vi "S8300E_SATA_IF_TEST_WIH.vi"() -> ()   [LabVIEW 2011]
panel:
  out "PRELOG2":string
  out "PRELOG1":string
  out "SATA_HDD_SIZE":string
  out "CMDList":cluster{string, string, string}[](array[cluster])
  out "log msg":string
  out "VISA resource name out":refnum<visa-resource-name>
  out "BEGIN TIME":u32
  out "進行狀況":string
  # "2015-6-1"
  # "S8300E SATA Interface Test(接UART COM9)"
  # "Error Code:SATA-IF"
  # "Step1:Check SATA HDD Size\nStep2:Check SATA HDD Interface"
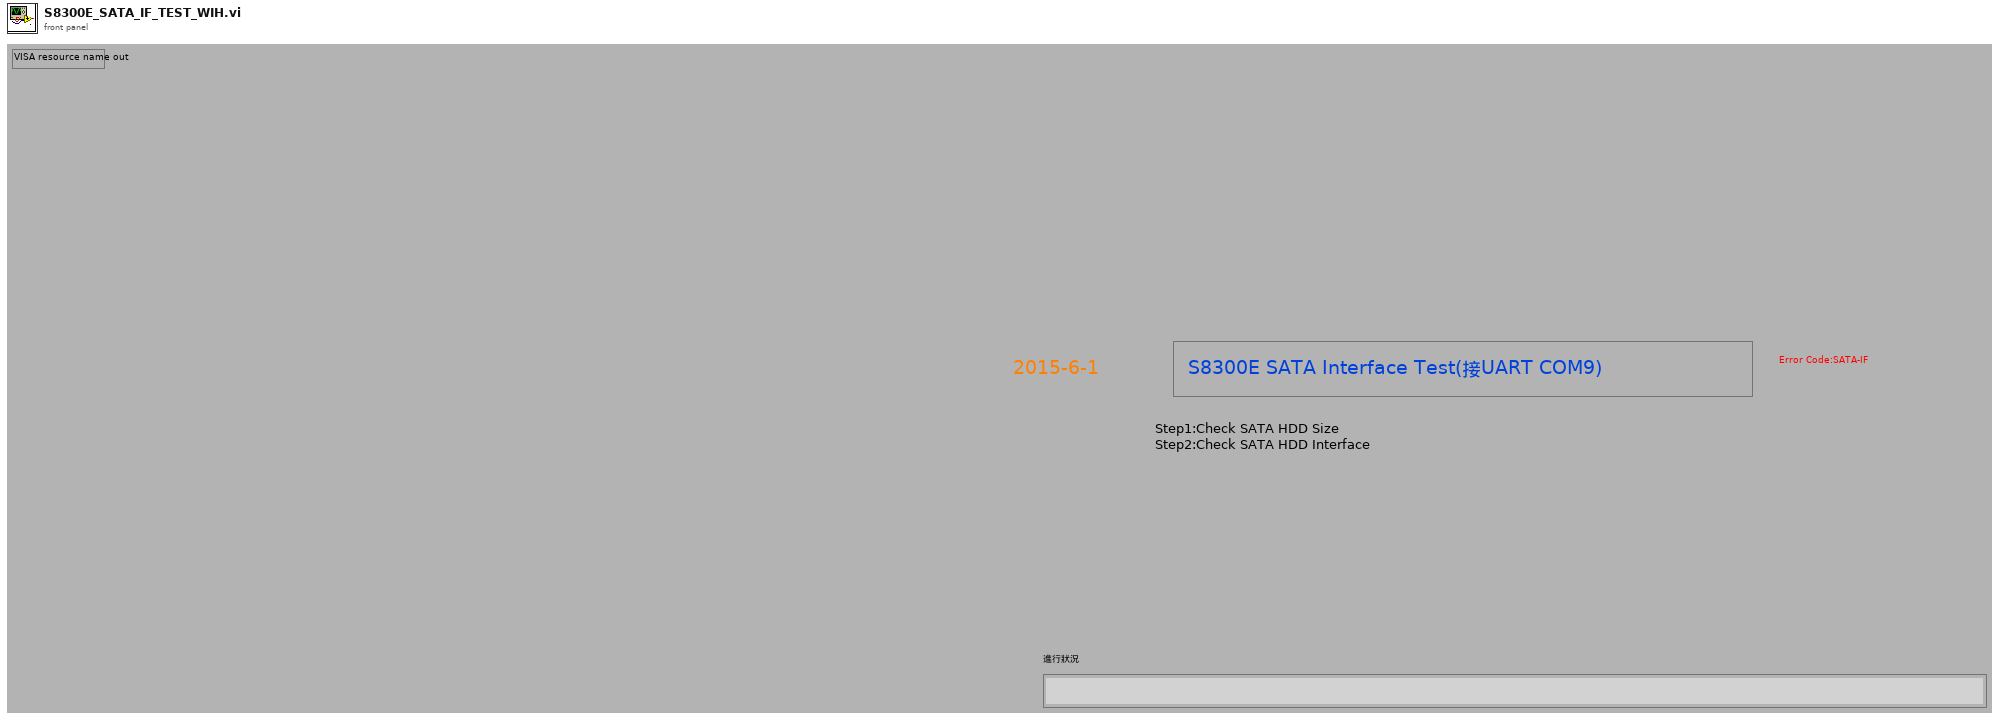
[diagram p1: front panel]
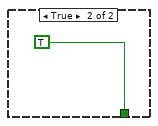
[diagram p7: hidden frame]
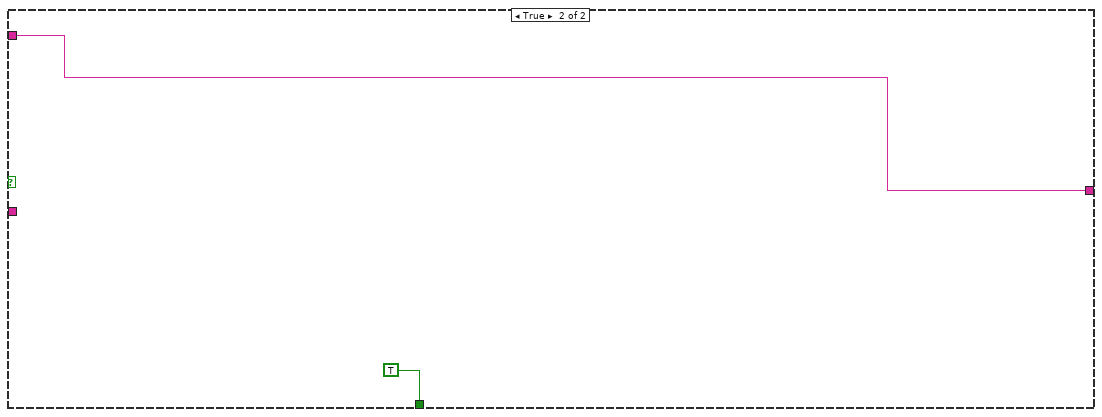
[diagram p9: hidden frame]
diagram:
  n1 = flat-sequence {
    frame #0 {
      n2 = Tick Count (ms)() -> (millisecond timer value=→"BEGIN TIME":u32)
    }
    frame #1 {
      n3 = property on="進行狀況" class="Str"("Blinking"=TRUE) -> ()  [unwired: 2 in, 2 out]
      "進行狀況" <- "進入測試準備中...." ("進行狀況")
    }
    frame #2 {
      n4 = call "SUB_SearchFile_inFolder.vi"("Search Filename in Folder"="S8300E_sfcs_misc.txt") -> ("File Existing True/Flase"=w4:bool)  [unwired: 1 in]
      n5 = case shown="False" w4 {
        frame False {
          n6 = flat-sequence {
            frame #0 {
              n7 = call "Display Message to User"() -> ()  [unwired: 10 in, 2 out]
            }
            frame #1 {
              n8 = call "SUB_Writelog.vi"("Pass/Fail"="Fail:S8300E_SATA_IF_TEST") -> ()  [unwired: 2 in]
            }
            frame #2 {
              n9 = Quit LabVIEW(quit? (T)=TRUE) -> ()
            }
          }
        }
        frame True {
        }
      }
    }
    frame #3 {
      n10 = call "SUB_Read_specifFile.vi"("name or relative path"="S8300E_sfcs_misc.txt" ("Search Filename in Folder")) -> ("text"=w11:string)  [unwired: 1 in, 1 out]
      n11 = call "SUB_FindSpecificString.vi"("Find this String"="UUT_SATA_HDD_SZIE=", "String data"=w11) -> ("before \"; \" string"=→"SATA_HDD_SIZE":string, "Found"=w9:bool)  [unwired: 2 in]
      n12 = case shown="False" w9 {
        frame False {
          n13 = flat-sequence {
            frame #0 {
              n14 = call "Display Message to User2"() -> ()  [unwired: 10 in, 2 out]
            }
            frame #1 {
              n15 = call "SUB_Writelog.vi"("Pass/Fail"="Fail:S8300E_SATA_IF_TEST") -> ()  [unwired: 2 in]
            }
            frame #2 {
              n16 = Quit LabVIEW(quit? (T)=TRUE) -> ()
            }
          }
        }
        frame True {
        }
      }
    }
    frame #4 {
      n17 = local read "SATA_HDD_SIZE"() -> (w21:string)
      n18 = Concatenate Strings("PASSED=", w21) -> (w20:string)
      n19 = Concatenate Strings("./sata.sh -s 1", "\r") -> (w26:string)
      n20 = Concatenate Strings("./sata.sh -t 1", "\r") -> (w17:string)
      n21 = Bundle(w17, "PASSED", "Checking SATA  HDD Interface") -> ()  [unwired: 1 in, 1 out]
      n22 = Bundle(w26, w20, "Checking SATA  HDD Size") -> (w24:cluster{string, string, string})  [unwired: 1 in]
      n23 = Build Array(w24) -> (→"CMDList":cluster{string, string, string}[])
    }
    frame #5 {
      n24 = call "SUB_COM1_CLOSE.vi"("VISA resource name"=refnum<visa-resource-name> "COM9") -> ()  [unwired: 3 in]
    }
    frame #6 {
      n25 = case shown="True" TRUE {
        frame False {
        }
        frame True {
          w32 = "\r"
          n26 = call "SUB_COM9_INIT.vi"("baud rate"=u32 115200) -> ("VISA resource name out"=w36:refnum<visa-resource-name>)  [unwired: 1 in, 1 out]
          "VISA resource name out" <- w36
          n27 = Concatenate Strings(w32, w32, w32) -> (w31:string)
          n28 = call "SUB_COM1Wrt.vi"("VISA resource name"=w36, "write buffer"=w31) -> ("duplicate VISA resource name"=w33:refnum<visa-resource-name>)  [unwired: 1 in, 1 out]
          n29 = call "SUB_ContinueCom1Read.vi"("Numeric"=1200, "duplicate VISA resource name 2"=w33) -> ()  [unwired: 1 in, 3 out]
        }
      }
    }
    frame #7 {
      n30 = case shown="True" TRUE {
        frame False {
        }
        frame True {
          n31 = while {
            stop <- w49 stop-if-true
            w44 = "s8300e_func_test#" ("Find this String")
            w41 = "\r"
            n32 = local read "VISA resource name out"() -> (w39:refnum<visa-resource-name>)
            n33 = Concatenate Strings(w41, w41, w41) -> (w42:string)
            n34 = call "SUB_ContinueCom1Read.vi"("Numeric"=1200, "duplicate VISA resource name 2"=w39) -> ("duplicate VISA resource name"=w38:refnum<visa-resource-name>)  [unwired: 1 in, 2 out]
            n35 = Tick Count (ms)() -> (millisecond timer value=w47:u32)
            n36 = call "SUB_COM1Wrt.vi"("VISA resource name"=w38, "write buffer"=w42) -> ("duplicate VISA resource name"=w48:refnum<visa-resource-name>)  [unwired: 1 in, 1 out]
            n37 = call "SUB_READ_COM1_FindString_timeout.vi"("Find this String"=w44, "Timeout Seccond"=3.0, "Begin time"=w47, "duplicate VISA resource name 2"=w48) -> ("Output String"=w45:string)  [unwired: 1 in, 2 out]
            n38 = call "SUB_FindSpecificString.vi"("Find this String"=w44, "String data"=w45) -> ("Found"=w43:bool)  [unwired: 2 in, 1 out]
            n39 = case shown="False" w43 {
              tunnel: [w54 TRUE] -> w49
              tunnel: w45 -> [w51 _]
              frame False {
                w53 = "UART無正確反應!需有S8300E字串" ("Status")
                n40 = call "SUB_YESNO.vi"("Debug View"=w51, "Status"=w53) -> ("yes/no"=w57:enum32{"No Selection", "Yes", "No", "None"})  [unwired: 1 in]
                n41 = Concatenate Strings(w53, "\n", w51) -> (w50:string)
                n42 = Equal?(x=w57, y=enum32{"No Selection", "Yes", "No", "None"}."No") -> (x = y?=w55:bool)
                n43 = case shown="True" w55 {
                  tunnel: [_ w59] -> w54
                  tunnel: w50 -> [_ w58]
                  frame False {
                  }
                  frame True {
                    n44 = flat-sequence {
                      tunnel: w58 -> [w60]
                      tunnel: [w66] -> w59
                      frame #0 {
                        n45 = Concatenate Strings("Fail:S8300E_SATA_IF_TEST" ("Pass/Fail"), "\n", w60) -> (w61:string)
                        n46 = call "SUB_Writelog.vi"("Pass/Fail"=w61) -> ()  [unwired: 2 in]
                      }
                      frame #1 {
                        n47 = call "SUB_SFCS_SendResult.vi"("ErrorCode"="UART", "PASS_Fail (1/0)"=i8 0) -> ()  [unwired: 1 out]
                      }
                      frame #2 {
                        w66 = TRUE ("quit? (T)")
                        n48 = Quit LabVIEW(quit? (T)=w66) -> ()
                      }
                    }
                  }
                }
              }
              frame True {
              }
            }
          }
        }
      }
    }
    frame #8 {
      n49 = local read "CMDList"() -> (w68:cluster{string, string, string}[])
      n50 = Array Size(array=w68) -> (size(s)=w71:i32)
      n51 = for {
        N: w71 -> [_]
        shift-right: [w74] -> w69
        shift-left: "" -> [w72]
        i -> [w76]
        n52 = while {
          tunnel: w76 -> [w94]
          shift-right: [w83] -> w75
          shift-left: "" -> [w82]
          stop <- w88 stop-if-true
          n53 = local read "VISA resource name out"() -> (w90:refnum<visa-resource-name>)
          n54 = local read "CMDList"() -> (w86:cluster{string, string, string}[])
          n55 = Index Array(array=w86, index=w94) -> (element=w87:cluster{string, string, string})
          n56 = Unbundle(w87) -> (w81:string, w84:string, w85:string)
          n57 = call "SUB_COM1Wrt.vi"("VISA resource name"=w90, "write buffer"=w81) -> ("duplicate VISA resource name"=w93:refnum<visa-resource-name>)  [unwired: 1 in, 1 out]
          n58 = Tick Count (ms)() -> (millisecond timer value=w92:u32)
          n59 = call "SUB_READ_COM1_FindString_timeout.vi"("Find this String"=w84, "Timeout Seccond"=2.0, "Begin time"=w92, "duplicate VISA resource name 2"=w93) -> ("Output String"=w79:string, "Found String"=w89:bool)  [unwired: 1 in, 1 out]
          n60 = Concatenate Strings(w81, "\n", w79) -> (w77:string)
          n61 = local write "進行狀況"(w85) -> ()
          n62 = case shown="False" w89 {
            tunnel: [_ TRUE] -> w88
            tunnel: w79 -> [w98 _]
            tunnel: [w96 w114] -> w78
            tunnel: w77 -> [w97 w114]
            frame False {
              w100 = "SATA測試失敗!有接SATA DRIVE" ("string")
              n63 = call "SUB_YESNO.vi"("Debug View"=w98, "Status"=w100) -> ("yes/no"=w103:enum32{"No Selection", "Yes", "No", "None"})  [unwired: 1 in]
              n64 = Concatenate Strings(w100, "\n", w97) -> (w95:string)
              n65 = Equal?(x=w103, y=enum32{"No Selection", "Yes", "No", "None"}."No") -> (x = y?=w101:bool)
              n66 = case shown="True" w101 {
                tunnel: [w104 _] -> w96
                tunnel: w95 -> [w104 w105]
                frame False {
                }
                frame True {
                  n67 = flat-sequence {
                    tunnel: w105 -> [w106]
                    frame #0 {
                      w108 = "\n"
                      n68 = local read "PRELOG2"() -> (w110:string)
                      n69 = local read "PRELOG1"() -> (w109:string)
                      n70 = Concatenate Strings("Fail:S8300E_SATA_IF_TEST" ("Pass/Fail"), w108, w110, w108, w109, w108, w106) -> (w107:string)
                      n71 = call "SUB_Writelog.vi"("Pass/Fail"=w107) -> ()  [unwired: 2 in]
                    }
                    frame #1 {
                      n72 = call "SUB_SFCS_SendResult.vi"("PASS_Fail (1/0)"=i8 0) -> ()  [unwired: 1 in, 1 out]
                    }
                    frame #2 {
                      n73 = Quit LabVIEW(quit? (T)=TRUE) -> ()
                    }
                  }
                }
              }
            }
            frame True {
            }
          }
          n74 = Concatenate Strings(w82, w78) -> (w83:string)
          "PRELOG1" <- w83
        }
        n75 = Concatenate Strings(w72, w75) -> (w74:string)
        "PRELOG2" <- w74
      }
      "log msg" <- w69
    }
    frame #9 {
      n76 = call "SUB_COM1_CLOSE.vi"("VISA resource name"=refnum<visa-resource-name> "COM9") -> ()  [unwired: 3 in]
    }
    frame #10 {
      w119 = "***Not Good ***" ("replace string (\"\")")
      n77 = local read "log msg"() -> (w123:string)
      n78 = local read "BEGIN TIME"() -> (w128:u32)
      n79 = Tick Count (ms)() -> (millisecond timer value=w127:u32)
      n80 = call "SUB_CAL_TESTTIME.vi"("Test Item name"="S8300E_SATA_IF_TEST", "Stop tick time"=w127, "Start tick time"=w128) -> ("Test Time output"=w125:string)  [unwired: 2 in]
      n81 = Concatenate Strings("Pass:S8300E_SATA_IF_TEST", "\n", w123, w125) -> (w118:string)
      n82 = call "SUB_SEARCH_REPLACE_STR.vi"("replace string (\"\")"=w119, "search string"="FAILED", "input string"=w118) -> ("result string"=w121:string)  [unwired: 2 in]
      n83 = call "SUB_SEARCH_REPLACE_STR.vi"("replace string (\"\")"=w119, "search string"="FAIL", "input string"=w121) -> ("result string"=w117:string)  [unwired: 2 in]
      n84 = call "SUB_Writelog.vi"("Pass/Fail"=w117) -> ()  [unwired: 2 in]
    }
    frame #11 {
      n85 = Request Deallocation(TRUE ("flag")) -> ()
    }
    frame #12 {
      n86 = Quit LabVIEW(quit? (T)=TRUE ("stop? (T)")) -> ()
    }
  }
